vi "Configuration - Load.vi"(8 "error in (no error)":errorcluster, 11 "Configuration Data":T1) -> (0 "error out":errorcluster, 3 "Configuration Data":T1)   [LabVIEW 2017]
doc: "Reads configuration data from the external TDMS file"
uses:
  Controls/ConfigData.ctl
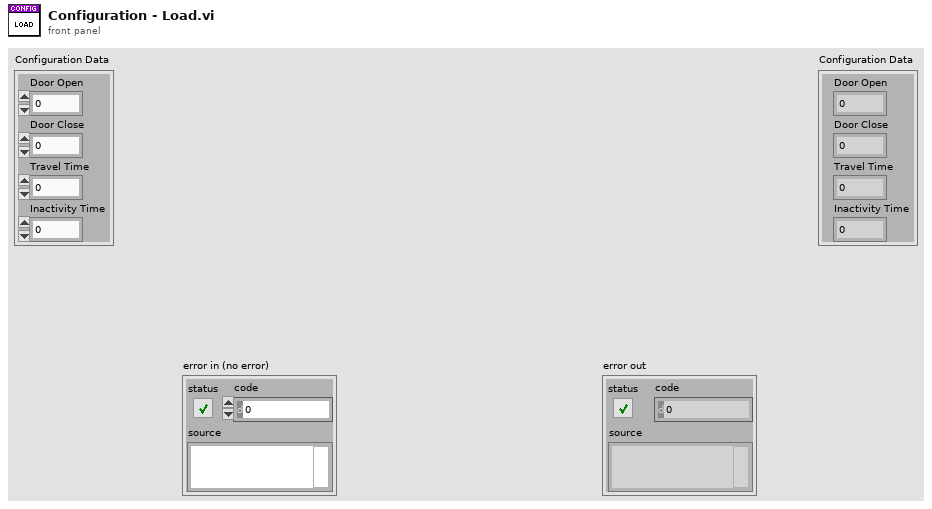
[diagram p1: front panel]
types:
  T1 = typedef "ConfigData.ctl" = cluster{"Door Open":dbl, "Door Close":dbl, "Travel Time":dbl, "Inactivity Time":dbl}
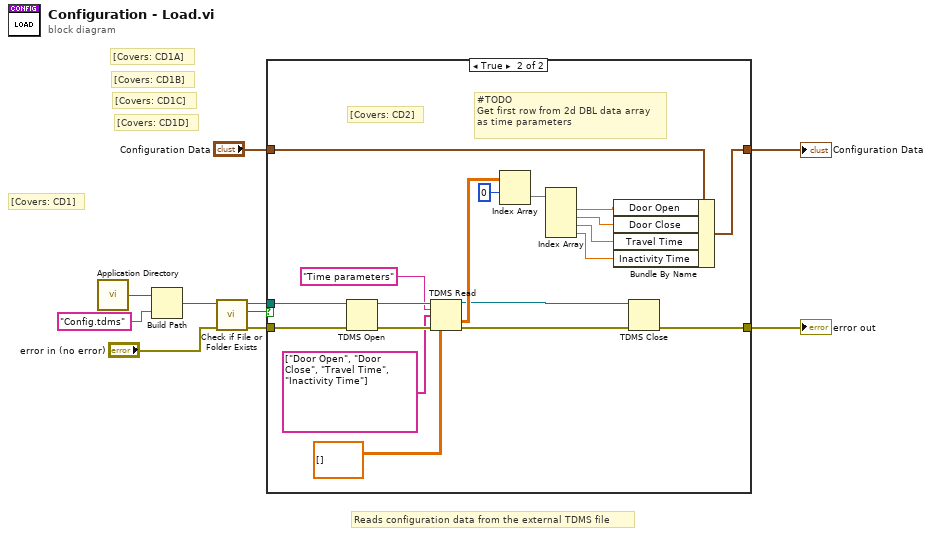
[diagram p0: block diagram]
diagram:
  # "[Covers: CD1D]"
  # "[Covers: CD1C]"
  # "[Covers: CD1B]"
  # "[Covers: CD1A]"
  # "[Covers: CD1]"
  # "Reads configuration data from the external TDMS file"
  n1 = call <vilib>:"Application Directory.vi"() -> ("Application Directory"=w10:path)
  n2 = Build Path(base path=w10, name or relative path="Config.tdms") -> (appended path=w8:path)
  n3 = call <vilib>:"Check if File or Folder Exists.vi"("error in (no error)"="error in (no error)", "path"=w8) -> ("error out"=w4:errorcluster, "file or folder exists?"=w6:bool, "dup path"=w5:path)  [unwired: 7 in]
  n4 = case shown="True" w6 {
    tunnel: w5 -> [_ w30]
    tunnel: w4 -> [w12 w31]
    tunnel: [w12 w13] -> w3
    tunnel: "Configuration Data" -> [w11 w21]
    tunnel: [w11 w16] -> w1
    frame False {
      # "Create new config file and write default changes"
      # "[Covers: CD3]"
    }
    frame True {
      # "#TODO\nGet first row from 2d DBL data array\nas time parameters"
      # "[Covers: CD2]"
      n5 = TDMS Open(8:w31, 11:w30) -> (0:w29:errorcluster, 3:w28:refnum<k34>)  [unwired: 5 in]
      n6 = TDMS Read(0:w28, 5:"Time parameters" ("group name in"), 7:string[] ["Door Open", "Door Close", "Travel Time", "Inactivity Time"], 11:w29, 12:dbl[][] []) -> (4:w15:refnum<k34>, 10:w24:dbl[][], 15:w14:errorcluster)  [unwired: 3 in, 3 out]
      n7 = Index Array(array=w24, index (row)=0) -> (element=w22:dbl[])  [unwired: 1 in]
      n8 = Index Array(array=w22) -> (element #1=w20:dbl, element #2=w19:dbl, element #3=w18:dbl, element #4=w17:dbl)  [unwired: 4 in]
      n9 = Bundle By Name(cluster=w21, "Door Open"=w20, "Door Close"=w19, "Travel Time"=w18, "Inactivity Time"=w17) -> (w16:T1)
      n10 = TDMS Close(8:w14, 11:w15) -> (0:w13:errorcluster)  [unwired: 1 out]
    }
  }
  "Configuration Data" <- w1
  "error out" <- w3
